vi "Configure Session.vi"(8 "error in":errorcluster, 11 "Plugin in":refnum<class "StreamReader.lvclass">) -> (0 "error out":errorcluster, 3 "Plugin out":refnum<class "StreamReader.lvclass">)   [LabVIEW 2024, in "StreamReader.lvlib" / "StreamReader.lvclass"]
uses:
  StreamReader.lvclass
  C:/Program Files/National Instruments/LabVIEW 2024/vi.lib/FlexLogger/SDK/PluginSDK.lvlibp/PEFClasses/SDK/Plugin/Plugin.lvclass
  StreamReader.lvclass/StreamReader.ctl
  StreamReader Strings.vi
  <vilib>/FlexLogger/SDK/PluginSDK.lvlibp/PEFClasses/SDK/Plugin/ParameterAccess/Read String.vi
  <vilib>/FlexLogger/SDK/PluginSDK.lvlibp/PEFClasses/SDK/Plugin/ParameterAccess/Read I32.vi
  <vilib>/FlexLogger/SDK/PluginSDK.lvlibp/PEFClasses/SDK/Plugin/Plugin.lvclass
  <vilib>/FlexLogger/SDK/PluginSDK.lvlibp
  C:/Program Files/National Instruments/LabVIEW 2024/vi.lib/FlexLogger/SDK/PluginSDK.lvlibp/PEFClasses/SDK/Processing Element/Processing Element.lvclass
  C:/dev/niflexlogger-plugins/plugins/StreamReader/source/StreamReader/StreamReader.lvclass
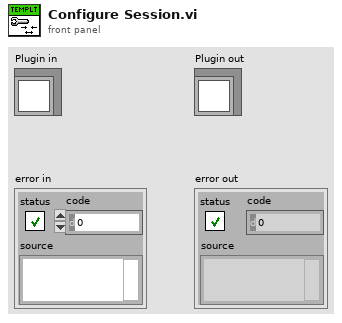
[diagram p1: front panel]
types:
  T1 = typedef "StreamReader.lvlib/StreamReader.lvclass/StreamReader Parameters.ctl" = cluster{"Reader URL":string, "Writer URL":string, "Buffer Size":i32, "Reader endpoint":refnum<k21>, "Channel Names":string[]}
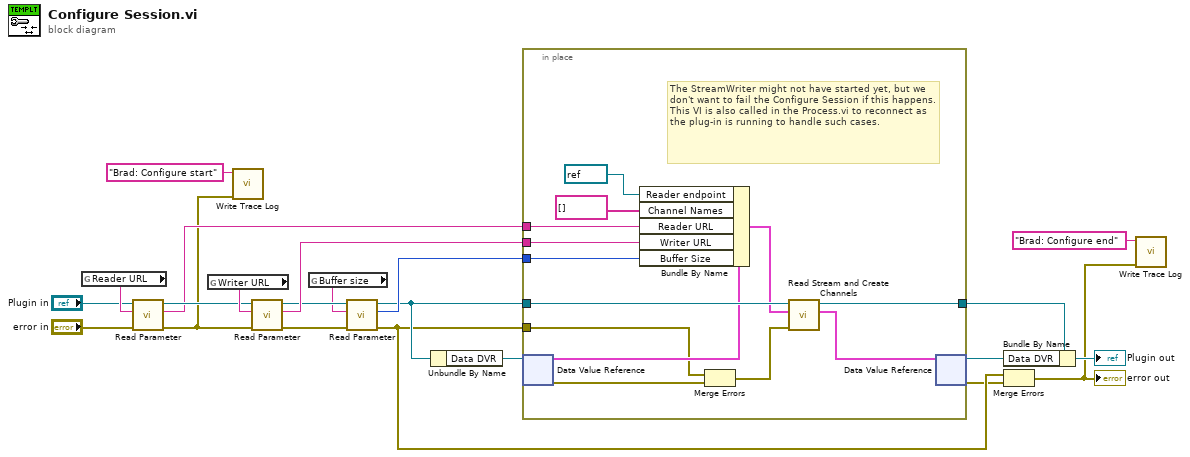
[diagram p0: block diagram]
diagram:
  n1 = global read "StreamReader Strings.vi" "Reader URL"() -> (w17:string)
  n2 = call-poly <vilib>:"Read Parameter.vi"("error in (no error)"="error in", "Name"=w17, "Plugin in"="Plugin in") -> ("error out"=w4:errorcluster, "Value"=w13:string, "Plugin out"=w15:refnum<class "StreamReader.lvclass">)  [unwired: 5 in, 1 out]
  n3 = global read "StreamReader Strings.vi" "Writer URL"() -> (w22:string)
  n4 = call <vilib>:"Write Trace Log.vi"("error in (no error)"=w4, "Message"="Brad: Configure start") -> ()  [unwired: 9 in, 1 out]
  n5 = call-poly <vilib>:"Read Parameter.vi"("error in (no error)"=w4, "Name"=w22, "Plugin in"=w15) -> ("error out"=w6:errorcluster, "Value"=w19:string, "Plugin out"=w7:refnum<class "StreamReader.lvclass">)  [unwired: 5 in, 1 out]
  n6 = global read "StreamReader Strings.vi" "Buffer size"() -> (w5:string)
  n7 = call-poly <vilib>:"Read Parameter.vi"("error in (no error)"=w6, "Name"=w5, "Plugin in"=w7) -> ("error out"=w9:errorcluster, "Value"=w20:i32, "Plugin out"=w12:refnum<class "StreamReader.lvclass">)  [unwired: 5 in, 1 out]
  n8 = Unbundle By Name(w12) -> ("Data DVR"=w11:refnum<data-value>)
  n9 = in-place {
    in-place-border: w20 -> [w35]
    in-place-border: w19 -> [w34]
    in-place-border: w12 -> [w33]
    in-place-border: [w31] -> w18
    in-place-border: w9 -> [w26]
    in-place-border: w13 -> [w30]
    # "The StreamWriter might not have started yet, but we don't want to fail the Configure Session if this happens.\nThis VI is also called in the Process.vi to reconnect as the plug-in is running to handle such cases."
    n10 = in-place-dvr #1(w11) -> (w29:T1, w27:errorcluster)
    n11 = Bundle By Name(cluster=w29, "Reader endpoint"=refnum<k21> refnum, "Channel Names"=string[] [], "Reader URL"=w30, "Writer URL"=w34, "Buffer Size"=w35) -> (w32:T1)
    n12 = Merge Errors(w26, w27) -> (w25:errorcluster)
    n13 = call-dynamic "Read Stream and Create Channels.vi"("error in (no error)"=w25, "StreamReader Parameters in"=w32, "Plugin in"=w33) -> ("StreamReader Parameters out"=w28:T1, "Plugin out"=w31:refnum<class "StreamReader.lvclass">)  [unwired: 5 in, 2 out]
    n14 = in-place-dvr #1(w28) -> (w10:refnum<data-value>, w8:errorcluster)
  }
  n15 = Bundle By Name(cluster=w18, "Data DVR"=w10) -> (→"Plugin out":refnum<class "StreamReader.lvclass">)
  n16 = Merge Errors(w9, w8) -> (w1:errorcluster)
  "error out" <- w1
  n17 = call <vilib>:"Write Trace Log.vi"("error in (no error)"=w1, "Message"="Brad: Configure end") -> ()  [unwired: 9 in, 1 out]
